vi "Compute Sample Length 2.vi"() -> (2 "Raw Smpl Len":i32)   [LabVIEW 2015, in "Tool Module.lvlib"]
uses:
  Tool Module.lvlib
  ToolModGLOB.vi
  Tool Config/Tool Cfg.lvlib
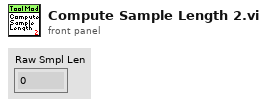
[diagram p1: front panel]
types:
  T1 = typedef "Tool Cfg.lvlib/_Tool Operation Config Cluster--typedef.ctl" = cluster{"Use Tool Cfg":bool, "Use Tool Cal":bool, "Fake Data?":bool, "Mode":i16, "Array Subset Length":i16, "nArrays to Read":i16, "Full Array Read Length":i16, "nSubarrays/Sensor":i16}
  T2 = typedef "_Data Stream Fmt Params Cluster--typedef.ctl" = cluster{"Samples per Block":i32, "Raw Data Status Len":i32, "Fltr Data Status Len":i32}
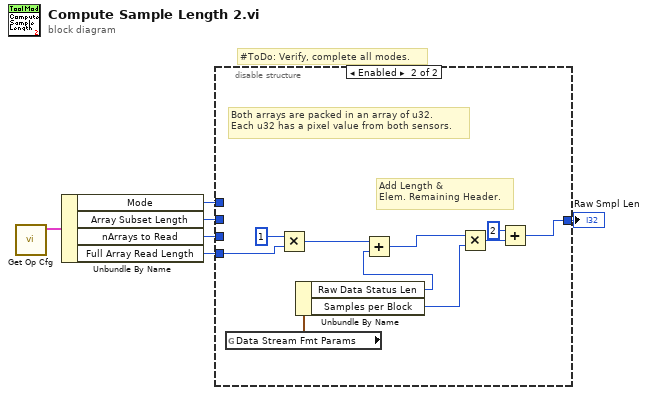
[diagram p0: block diagram]
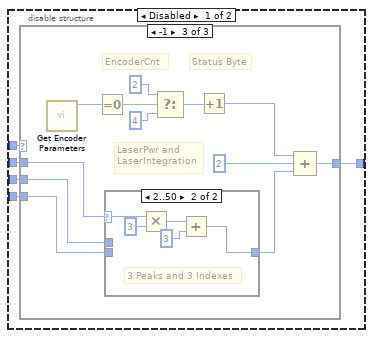
[diagram p2: hidden frame]
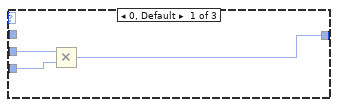
[diagram p3: hidden frame]
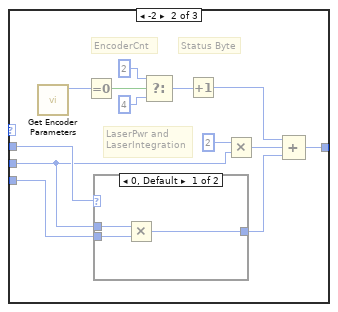
[diagram p4: hidden frame]
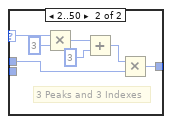
[diagram p5: hidden frame]
diagram:
  # "#ToDo: Verify, complete all modes."
  n1 = call "Get Op Cfg.vi"() -> ("Tool Operation Config"=w1:T1)  [unwired: 11 in]
  n2 = Unbundle By Name(w1) -> ("Mode"=w2:i16, "Array Subset Length"=w5:i16, "nArrays to Read"=w3:i16, "Full Array Read Length"=w4:i16)
  n3 = disable-structure shown="Enabled" {
    disable-tunnel: [w11 w58] -> w6
    disable-tunnel: w5 -> [w10 _]
    disable-tunnel: w4 -> [w9 w63]
    disable-tunnel: w3 -> [w8 _]
    disable-tunnel: w2 -> [w7 _]
    frame Disabled {
      n4 = case shown="-1" w7 {
        tunnel: w8 -> [w14 w20 w43]
        tunnel: w9 -> [w13 w21 w44]
        tunnel: w10 -> [_ w22 w45]
        tunnel: [w12 w17 w41] -> w11
        frame 0, Default {
          n5 = Multiply(x=w14, y=w13) -> (x*y=w12:i16)
        }
        frame -2 {
          # "LaserPwr and\nLaserIntegration"
          # "Status Byte"
          # "EncoderCnt"
          n6 = call "Get Encoder Parameters.vi"() -> ("Encoder Size"=w15:u16)  [unwired: 9 in, 2 out]
          n7 = Equal To 0?(x=w15) -> (x = 0?=w27:bool)
          n8 = case shown="0, Default" w22 {
            selector: w22 -> [_ w37]
            tunnel: w21 -> [w29 _]
            tunnel: w20 -> [w30 w32]
            tunnel: [w28 w31] -> w18
            frame 0, Default {
              n9 = Multiply(x=w30, y=w29) -> (x*y=w28:i16)
            }
            frame 2..50 {
              # "3 Peaks and 3 Indexes"
              n10 = Multiply(x=w37, y=i16 3) -> (x*y=w35:i16)
              n11 = Add(x=w35, y=i16 3) -> (x+y=w33:i16)
              n12 = Multiply(x=w33, y=w32) -> (x*y=w31:i16)
            }
          }
          n13 = Select(t=2 ("Raw Smpl Len"), s=w27, f=4 ("Raw Smpl Len")) -> (s? t:f=w24:i32)
          n14 = Increment(x=w24) -> (x+1=w16:i32)
          n15 = Multiply(x=2 ("Raw Smpl Len"), y=w20) -> (x*y=w19:i32)
          n16 = Compound Arithmetic op=ADD(w16, w19, w18) -> (w17:i32)
        }
        frame -1 {
          # "LaserPwr and\nLaserIntegration"
          # "Status Byte"
          # "EncoderCnt"
          n17 = call "Get Encoder Parameters.vi"() -> ("Encoder Size"=w38:u16)  [unwired: 9 in, 2 out]
          n18 = Equal To 0?(x=w38) -> (x = 0?=w49:bool)
          n19 = case shown="2..50" w45 {
            selector: w45 -> [_ w55]
            tunnel: w44 -> [w50 _]
            tunnel: w43 -> [_ _]
            tunnel: [w50 w51] -> w42
            frame 0, Default {
            }
            frame 2..50 {
              # "3 Peaks and 3 Indexes"
              n20 = Multiply(x=w55, y=i16 3) -> (x*y=w53:i16)
              n21 = Add(x=w53, y=i16 3) -> (x+y=w51:i16)
            }
          }
          n22 = Select(t=2 ("Raw Smpl Len"), s=w49, f=4 ("Raw Smpl Len")) -> (s? t:f=w46:i32)
          n23 = Increment(x=w46) -> (x+1=w40:i32)
          n24 = Compound Arithmetic op=ADD(w40, 2 ("Raw Smpl Len"), w42) -> (w41:i32)
        }
      }
    }
    frame Enabled {
      # "Add Length & \nElem. Remaining Header."
      # "Both arrays are packed in an array of u32.\nEach u32 has a pixel value from both sensors."
      n25 = global read "ToolModGLOB.vi" "Data Stream Fmt Params"() -> (w65:T2)
      n26 = Multiply(x=i16 1 ("y"), y=w63) -> (x*y=w56:i16)
      n27 = Unbundle By Name(w65) -> ("Raw Data Status Len"=w64:i32, "Samples per Block"=w61:i32)
      n28 = Add(x=w56, y=w64) -> (x+y=w62:i32)
      n29 = Multiply(x=w62, y=w61) -> (x*y=w60:i32)
      n30 = Add(x=2, y=w60) -> (x+y=w58:i32)
    }
  }
  "Raw Smpl Len" <- w6
